vi "Max uncompressed size.vi"(8 "error in (no error)":errorcluster, 10 "srcHandle":string) -> (0 "error out":errorcluster, 2 "uncompressed size":i32)   [LabVIEW 2020, in "lvzstd.lvlib"]
uses:
  lvzstd.lvlib
  Private/Path FGV.vi
  <vilib>/Utility/error.llb/Error Cluster From Error Code.vi
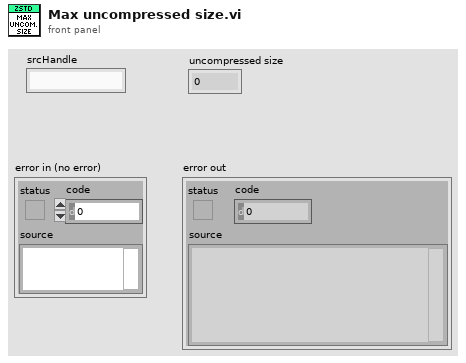
[diagram p1: front panel]
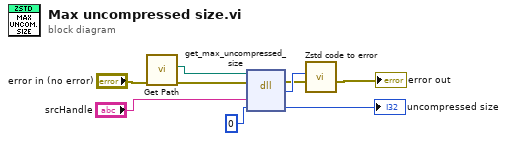
[diagram p0: block diagram]
diagram:
  n1 = call "Get Path.vi"("error in (no error)"="error in (no error)") -> ("error out (no error)"=w2:errorcluster, "Library Path"=w1:path)  [unwired: 9 in]
  n2 = dll-call lib="?" fn="get_max_uncompressed_size"(path in=w1, error in=w2, "srcHandle"="srcHandle", "uncompressed_size"=0 ("max_compressed_size")) -> (error out=w4:errorcluster, "error_code"=w6:i32, "uncompressed_size"=→"uncompressed size":i32)  [unwired: 2 in, 1 out]
  n3 = call "Zstd code to error.vi"("error in"=w4, "Error code"=w6) -> ("error in (no error)"=→"error out":errorcluster)  [unwired: 9 in]
